vi "SerialCommunicationFGV.vi"(7 "ctl":T1(ring), 8 "errorIn":errorcluster caption="error out", 9 "bufferWrite":string, 10 "visaResourceNameIn":refnum<visa-resource-name>) -> (0 "errorOut":errorcluster caption="error out", 1 "bufferRead":string, 2 "VISA resource name out":refnum<visa-resource-name>)   [LabVIEW 2023]
uses:
  b791345b-9e7b-4b80-9c90-3f668f179418.vi
  7c134577-f2c4-43c6-8360-c51b04b89414.vi
  <vilib>/Instr/_visa.llb/VISA Configure Serial Port (Instr).vi
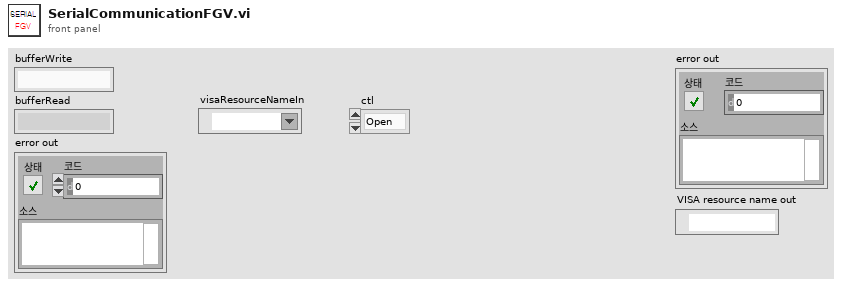
[diagram p1: front panel]
types:
  T1 = enum16{"Open", "Write Only", "Read Only", "Write&Read", "Close"}
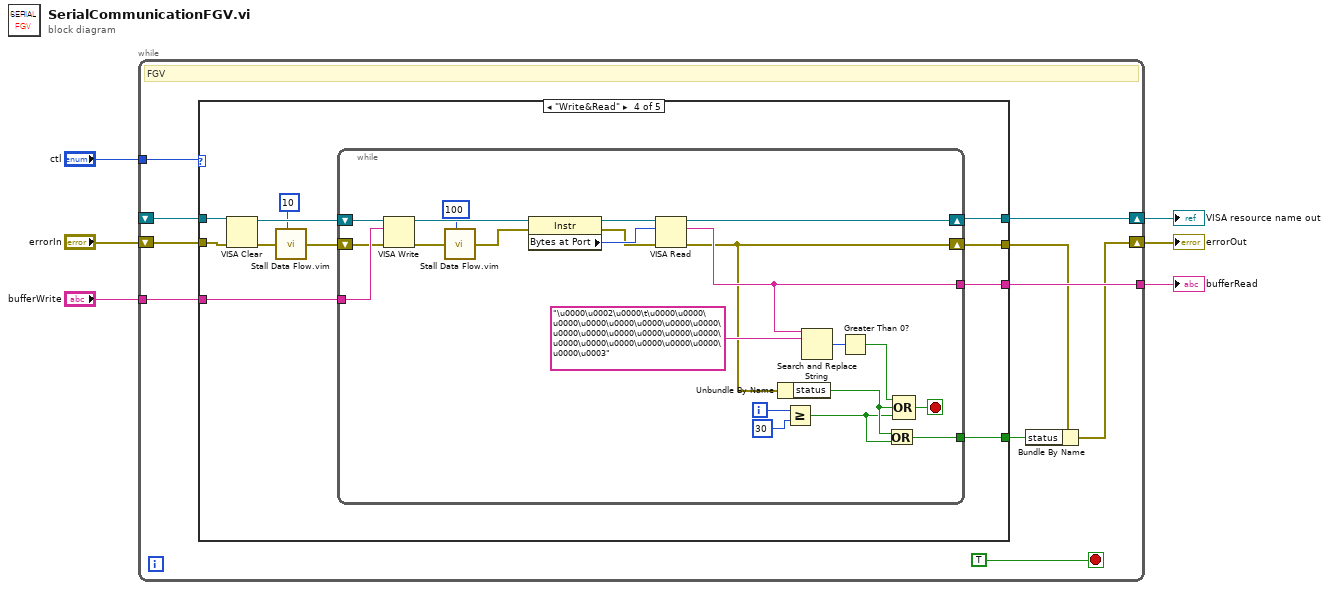
[diagram p0: block diagram]
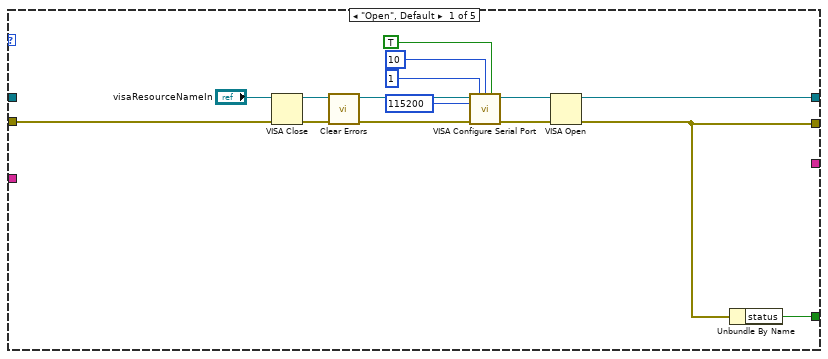
[diagram p2: hidden frame]
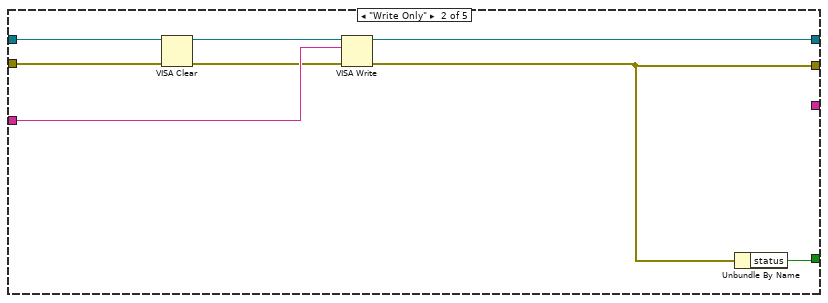
[diagram p3: hidden frame]
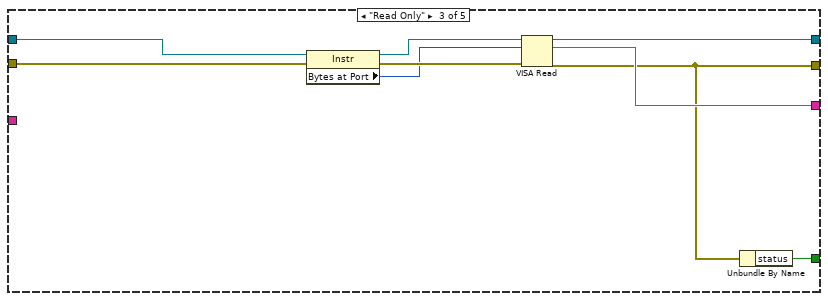
[diagram p4: hidden frame]
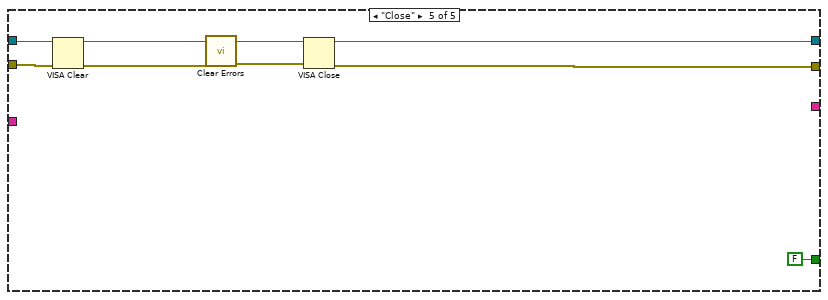
[diagram p5: hidden frame]
diagram:
  n1 = while {
    tunnel: "ctl" -> [w16]
    shift-right: [w15] -> w1
    shift-left: _ -> [w14]
    shift-right: [w8] -> w2
    shift-left: "errorIn" -> [w13]
    tunnel: "bufferWrite" -> [w11]
    tunnel: [w10] -> w4
    stop <- TRUE stop-if-true
    # "FGV"
    n2 = case shown="\"Write&Read\"" w16 {
      tunnel: [w24 w36 w46 w57 w81] -> w15
      tunnel: [w18 w30 w39 w48 w82] -> w9
      tunnel: w14 -> [_ w37 w44 w53 w85]
      tunnel: w13 -> [w23 w33 w45 w52 w84]
      tunnel: w11 -> [_ w35 _ w51 _]
      tunnel: [_ _ w40 w56 _] -> w10
      tunnel: [w17 w31 w38 w47 FALSE ("status")] -> w7
      frame "Open", Default {
        n3 = VISA Close(VISA resource name="visaResourceNameIn", error in (no error)=w23) -> (error out=w25:errorcluster)
        n4 = call <vilib>:"Clear Errors.vi"("error in (no error)"=w25) -> ("error out"=w22:errorcluster)  [unwired: 5 in, 1 out]
        n5 = call-poly "VISA Configure Serial Port"("VISA resource name"="visaResourceNameIn", "timeout (10sec)"=u32 1, "termination char\n(0xA = '\\n' = LF)"=u8 10 ("termination char\n(0xA = '\\n' = LF)"), "Enable Termination\nChar (T)"=TRUE ("Enable Termination\nChar (T)"), "baud rate (9600)"=u32 115200, "error in (no error)"=w22) -> ("VISA resource name out"=w27:refnum<visa-resource-name>, "error out"=w26:errorcluster)  [unwired: 8 in]
        n6 = VISA Open(error in (no error)=w26, VISA resource name=w27) -> (VISA resource name=w24:refnum<visa-resource-name>, error out=w18:errorcluster)  [unwired: 3 in]
        n7 = Unbundle By Name(w18) -> ("status"=w17:bool)
      }
      frame "Write Only" {
        n8 = VISA Clear(VISA resource name=w37, error in (no error)=w33) -> (VISA resource name out=w34:refnum<visa-resource-name>, error out=w32:errorcluster)
        n9 = VISA Write(VISA resource name=w34, write buffer=w35, error in (no error)=w32) -> (VISA resource name out=w36:refnum<visa-resource-name>, error out=w30:errorcluster)  [unwired: 1 out]
        n10 = Unbundle By Name(w30) -> ("status"=w31:bool)
      }
      frame "Read Only" {
        n11 = property class="Instr"(reference=w44, error in=w45) -> (reference out=w43:refnum<visa-resource-name>, error out=w42:errorcluster, "Bytes at Port"=w41:u32)
        n12 = VISA Read(VISA resource name=w43, byte count=w41, error in (no error)=w42) -> (VISA resource name out=w46:refnum<visa-resource-name>, read buffer=w40:string, error out=w39:errorcluster)  [unwired: 1 out]
        n13 = Unbundle By Name(w39) -> ("status"=w38:bool)
      }
      frame "Write&Read" {
        n14 = VISA Clear(VISA resource name=w53, error in (no error)=w52) -> (VISA resource name out=w54:refnum<visa-resource-name>, error out=w55:errorcluster)
        n15 = call "Stall Data Flow.vim"("value in"=w55, "milliseconds to wait"=u32 10) -> ("value out"=w50:errorcluster)  [unwired: 1 out]
        n16 = while {
          tunnel: [w64] -> w56
          tunnel: w51 -> [w76]
          shift-right: [w79] -> w57
          shift-left: w54 -> [w78]
          shift-right: [w61] -> w48
          shift-left: w50 -> [w75]
          tunnel: [w58] -> w47
          i -> [w72]
          stop <- w74 stop-if-true
          n17 = VISA Write(VISA resource name=w78, write buffer=w76, error in (no error)=w75) -> (VISA resource name out=w77:refnum<visa-resource-name>, error out=w65:errorcluster)  [unwired: 1 out]
          n18 = call "Stall Data Flow.vim"("value in"=w65, "milliseconds to wait"=u32 100) -> ("value out"=w63:errorcluster)  [unwired: 1 out]
          n19 = property class="Instr"(reference=w77, error in=w63) -> (reference out=w69:refnum<visa-resource-name>, error out=w67:errorcluster, "Bytes at Port"=w68:u32)
          n20 = VISA Read(VISA resource name=w69, byte count=w68, error in (no error)=w67) -> (VISA resource name out=w79:refnum<visa-resource-name>, read buffer=w64:string, error out=w61:errorcluster)  [unwired: 1 out]
          n21 = Unbundle By Name(w61) -> ("status"=w60:bool)
          n22 = Greater Or Equal?(x=w72, y=30) -> (x >= y?=w59:bool)
          n23 = Search and Replace String(input string=w64, search string="\u0000\u0002\u0000\t\u0000\u0000\u0000\u0000\u0000\u0000\u0000\u0000\u0000\u0000\u0000\u0000\u0000\u0000\u0000\u0000\u0000\u0000\u0000\u0000\u0000\u0003" ("*(타입 *) &x")) -> (number of replacements=w71:i32)  [unwired: 6 in, 3 out]
          n24 = Greater Than 0?(x=w71) -> (x > 0?=w62:bool)
          n25 = Or(x=w60, y=w59) -> (x .or. y?=w58:bool)
          n26 = Compound Arithmetic op=OR ("복합 연산")(w62, w60, w59) -> (w74:bool)
        }
      }
      frame "Close" {
        n27 = VISA Clear(VISA resource name=w85, error in (no error)=w84) -> (VISA resource name out=w81:refnum<visa-resource-name>, error out=w83:errorcluster)
        n28 = call <vilib>:"Clear Errors.vi"("error in (no error)"=w83) -> ("error out"=w86:errorcluster)  [unwired: 5 in, 1 out]
        n29 = VISA Close(VISA resource name=w81, error in (no error)=w86) -> (error out=w82:errorcluster)
      }
    }
    n30 = Bundle By Name(cluster=w9, "status"=w7) -> (w8:errorcluster)
  }
  "bufferRead" <- w4
  "errorOut" <- w2
  "VISA resource name out" <- w1
